vi "read_ram_out.vi"() -> (3 "RAM_OUT":u8)   [LabVIEW 2015]
uses:
  <vilib>/rvi/eio/common/nirviEmuTemplateMethod_errors.vi
  <vilib>/eio/EIONode/EIONode.xnode
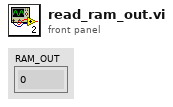
[diagram p1: front panel]
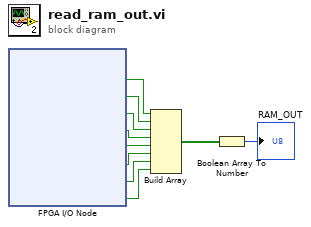
[diagram p0: block diagram]
diagram:
  n1 = xnode "FPGA I/O Node"() -> ("RAM_OUT[0]"=w10:bool, "RAM_OUT[1]"=w9:bool, "RAM_OUT[2]"=w8:bool, "RAM_OUT[3]"=w5:bool, "RAM_OUT[4]"=w4:bool, "RAM_OUT[5]"=w3:bool, "RAM_OUT[6]"=w1:bool, "RAM_OUT[7]"=w2:bool)  [unwired: 8 in, 8 out]
  n2 = Build Array(w10, w9, w8, w5, w4, w3, w1, w2) -> (w6:bool[])
  n3 = Boolean Array To Number(Boolean array=w6) -> (number=→"RAM_OUT":u8)
